vi "folder_check.vi"(8 "error in (no error)":errorcluster, 11 "stripped path":path) -> (0 "error out":errorcluster)   [LabVIEW 2015, in "ini_work_Library.lvlib"]
doc: "Created by Artem Shevelev\nshevelev.pro\nartem@shevelev.pro\nLabVIEW Portal: https://labviewportal.org/memberlist.php?mode=viewprofile&u=2340"
uses:
  ini_work_Library.lvlib
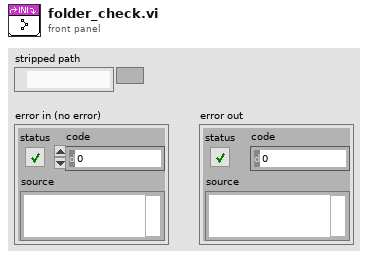
[diagram p1: front panel]
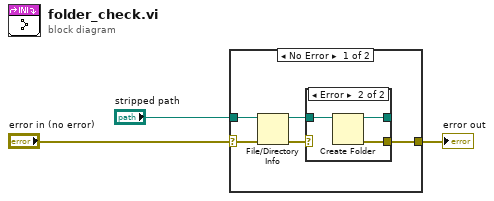
[diagram p0: block diagram]
diagram:
  n1 = case shown="No Error" "error in (no error)" {
    selector: "error in (no error)" -> [w4 w14]
    tunnel: [w8 w14] -> w3
    tunnel: "stripped path" -> [w7 _]
    frame No Error {
      n2 = File/Directory Info(path=w7, error in=w4) -> (path out=w6:path, error out=w5:errorcluster)  [unwired: 5 out]
      n3 = case shown="Error" w5 {
        selector: w5 -> [w9 _]
        tunnel: [w10 w12] -> _
        tunnel: w6 -> [w10 w13]
        tunnel: [w9 w11] -> w8
        frame No Error {
        }
        frame Error {
          n4 = Create Folder(path (use dialog)=w13) -> (created path=w12:path, error out=w11:errorcluster)  [unwired: 2 in, 1 out]
        }
      }
    }
    frame Error {
    }
  }
  "error out" <- w3
